vi "h5_close_file.vi"(8 "error in":errorcluster, 11 "h5 root ref":T1 format="%.0x") -> (0 "error out":errorcluster, 2 "ok?":bool, 3 "path":path)   [LabVIEW 2015]
doc: "This vi flushes the file, attempts to get it's path and the close it. Then, all the errors are cleared. <B>ok?</B> indicates whether the closing has been succesfull."
uses:
  <vilib>/addons/h5labview2/base/hid_t.ctl
  <vilib>/addons/h5labview2/file/H5F.lvlib
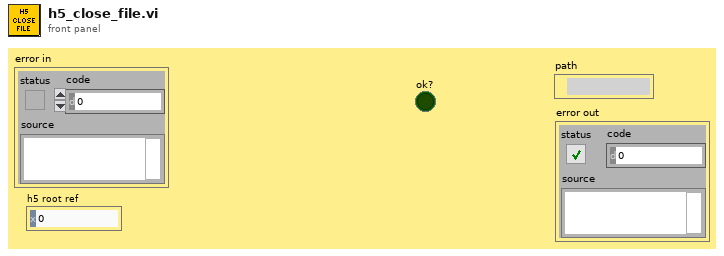
[diagram p1: front panel]
types:
  T1 = typedef "hid_t.ctl" = i32
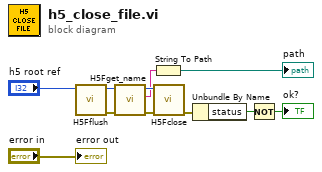
[diagram p0: block diagram]
diagram:
  n1 = call <vilib>:"H5Fflush.vi"("ref in"="h5 root ref") -> ("error out"=w2:errorcluster, "ref out"=w3:T1)  [unwired: 9 in]
  n2 = call <vilib>:"H5Fget_name.vi"("error in (no error)"=w2, "ref in"=w3) -> ("error out"=w7:errorcluster, "name"=w6:string, "ref out"=w8:T1)  [unwired: 7 in]
  n3 = String To Path(string=w6) -> (path=→"path":path)
  n4 = call <vilib>:"H5Fclose.vi"("error in (no error)"=w7, "ref"=w8) -> ("error out"=w5:errorcluster)  [unwired: 9 in]
  n5 = Unbundle By Name(w5) -> ("status"=w4:bool)
  n6 = Not(x=w4) -> (.not. x?=→"ok?":bool)
  "error out" <- "error in"
